vi "theta2_FRD.vi"(6 "freq unit":u16(ring) items=["Hz", "rad/s"], 7 "Sampling Time (s)":dbl=4e-05 format="%#_13g", 8 "error in (no error)":errorcluster, 9 "Data-name":string, 10 "freqs/omega":dbl[](array[numeric]), 11 "theta":dbl[](array[numeric])) -> (0 "error out":errorcluster, 3 "FRD-model":T1)   [LabVIEW 2017]
uses:
  controls/FrdData.ctl
  <vilib>/addons/Control Design/_Frequency Response Analysis/Frequency Response.llb/Frequency Response subVI/cd_Evaluate at Frequency (Zero-Pole-Gain).vi
  <vilib>/addons/Control Design/_Frequency Response Analysis/NI_CD_Frequency Response.lvlib
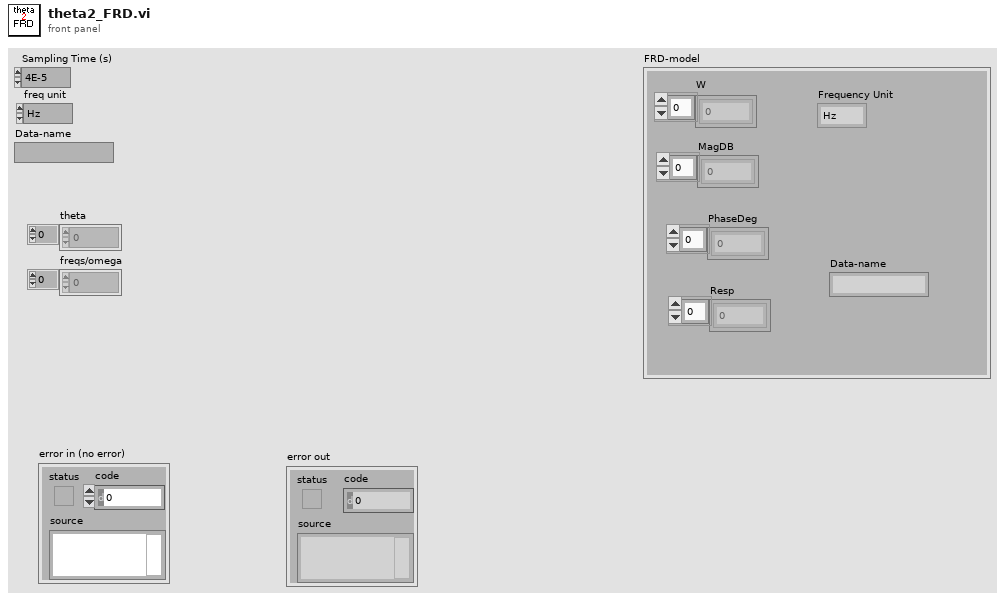
[diagram p1: front panel]
types:
  T1 = typedef "FrdData.ctl" = cluster{"Frequency Unit":enum16{"Hz", "rad/s"}, "W":dbl[], "MagDB":dbl[], "PhaseDeg":dbl[], "Resp":cdb[], "Data-name":string}
  T2 = typedef "NI_LinSys_Model Typedefs.lvlib/CD Zero-Pole-Gain Model (MIMO).ctl" = cluster{"properties":T3, "zero-pole-gain(s)":T4[][]}
  T3 = typedef "NI_LinSys_Model Typedefs.lvlib/CD General Elements.ctl" = cluster{"Model name":string, "Input names":string[], "Output names":string[], "Input Delays":dbl[], "Output Delays":dbl[], "Sampling Time":dbl, "Notes":string}
  T4 = typedef "NI_LinSys_Model Typedefs.lvlib/CD Zero-Pole-Gain Model (SISO).ctl" = cluster{"Gain":dbl, "Zeros":cdb[], "Poles":cdb[], "delay":dbl}
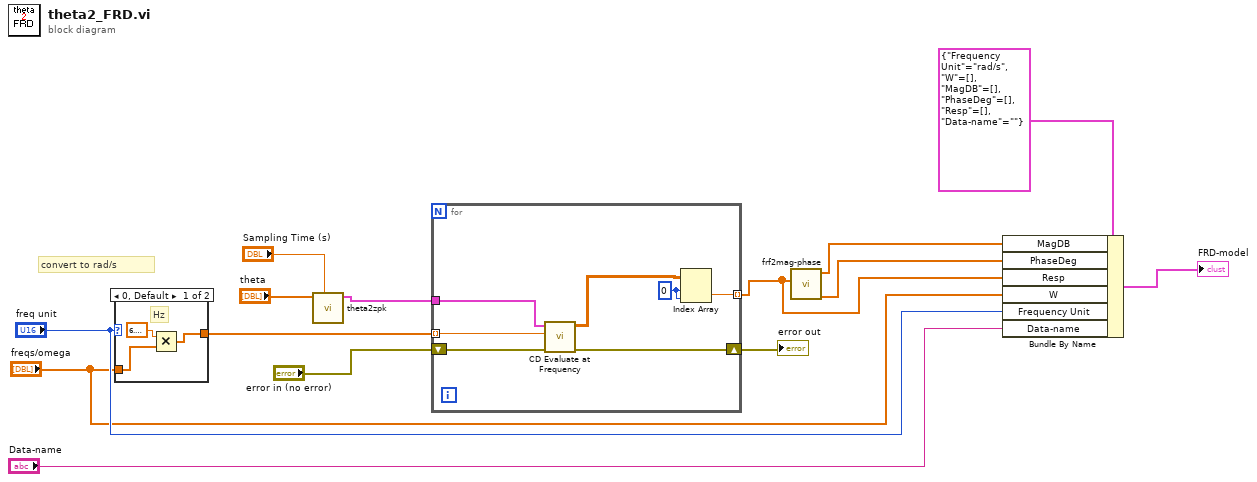
[diagram p0: block diagram]
diagram:
  # "convert to rad/s"
  n1 = case shown="0, Default" "freq unit" {
    tunnel: "freqs/omega" -> [w17 w18]
    tunnel: [w16 w18] -> w6
    frame 0, Default {
      # "Hz"
      n2 = Multiply(x=6.283185307179586, y=w17) -> (x*y=w16:dbl[])
    }
    frame 1 {
      # "rad/s"
    }
  }
  n3 = call "theta2zpk.vi"("Sampling Time (s)"="Sampling Time (s)", "theta in"="theta") -> ("Model Out"=w13:T2)  [unwired: 9 in]
  n4 = for {
    tunnel: w13 -> [w25]
    tunnel: w6 -> [w24] mode=indexing
    tunnel: [w21] -> w7 mode=indexing
    shift-right: [w19] -> w1
    shift-left: "error in (no error)" -> [w23]
    w22 = 0 ("index (row)")
    n5 = call-poly <vilib>:"CD Evaluate at Frequency.vi"("error in (no error)"=w23, "Frequency (rad/s)"=w24, "Zero-Pole-Gain Model"=w25) -> ("error out"=w19:errorcluster, "Response"=w20:cdb[][])  [unwired: 5 in, 2 out]
    n6 = Index Array(array=w20, index (row)=w22, index (col)=w22) -> (element=w21:cdb)
  }
  "error out" <- w1
  n7 = call "frf2mag-phase.vi"("G_frf"=w7) -> ("phase [deg]"=w8:dbl[], "mag-dB"=w9:dbl[])  [unwired: 9 in]
  n8 = Bundle By Name(cluster=T1 {"Frequency Unit"=enum."rad/s", "W"=[], "MagDB"=[], "PhaseDeg"=[], "Resp"=[], "Data-name"=""} ("FrdData Out 2"), "MagDB"=w9, "PhaseDeg"=w8, "Resp"=w7, "W"="freqs/omega", "Frequency Unit"="freq unit", "Data-name"="Data-name") -> (→"FRD-model":T1)
